vi "AcquisitionMVF_Reentrent.vi"(6 "error in":errorcluster, 7 "Session":T2, 9 "Image Rev":T1) -> (0 "camera error":errorcluster, 2 "Image Dst Out":T1, 3 "Acquisition OK?":bool)   [LabVIEW 2011]
uses:
  <vilib>/vision/Image Controls.llb/IMAQ Image.ctl
  <vilib>/userdefined/High Color/IMAQdx.ctl
  <vilib>/vision/NI_Vision_Development_Module.lvlib
  <vilib>/vision/driver/NI_Vision_Acquisition_Software.lvlib
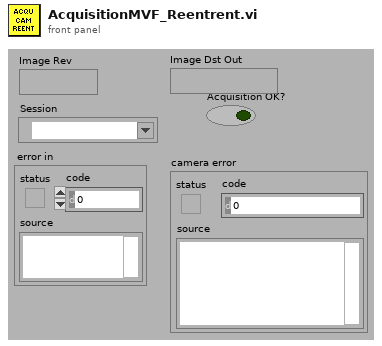
[diagram p1: front panel]
types:
  T1 = typedef "IMAQ Image.ctl" = refnum<image>
  T2 = typedef "IMAQdx.ctl" = refnum<k21>
  T3 = typedef "Image Type" = u32
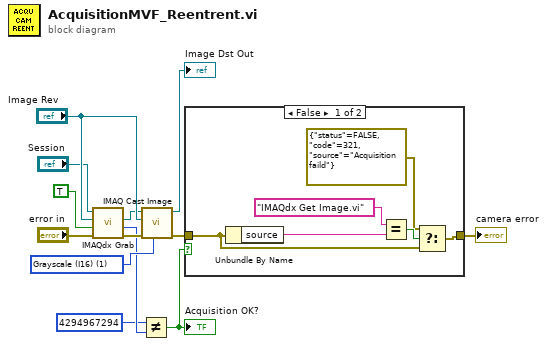
[diagram p0: block diagram]
diagram:
  w7 = T3 1 items=["Grayscale (U8)", "Grayscale (I16)", "Grayscale (SGL)", "Complex (CSG)", "RGB (U32)", "HSL (U32)", "RGB (U64)", "Grayscale (U16)"] ("Image Type")
  n1 = call <vilib>:"IMAQdx Grab.vi"("error in"="error in", "Wait for Next Buffer? (Yes)"=TRUE, "Image In"="Image Rev", "Session In"="Session") -> ("error out"=w6:errorcluster, "Buffer Number Out"=w3:u32, "Image Out"=w8:T1)  [unwired: 5 out]
  n2 = Not Equal?(x=u32 4294967294 ("Buffer Number Out"), y=w3) -> (x != y?=w13:bool)
  "Acquisition OK?" <- w13
  n3 = call "IMAQ Cast Image"("Image Type"=w7, "error in (no error)"=w6, "Image Dst"="Image Rev", "Image Src"=w8) -> ("error out"=w5:errorcluster, "Image Dst Out"=→"Image Dst Out":T1)  [unwired: 6 in]
  n4 = case shown="False" w13 {
    tunnel: w5 -> [w15 w20]
    tunnel: [w14 w20] -> w9
    frame False {
      n5 = Unbundle By Name(w15) -> ("source"=w19:string)
      n6 = Equal?(x="IMAQdx Get Image.vi", y=w19) -> (x = y?=w17:bool)
      n7 = Select(t=errorcluster {"status"=FALSE, "code"=321, "source"="Acquisition faild"} ("error in"), s=w17, f=w15) -> (s? t:f=w14:errorcluster)
    }
    frame True {
    }
  }
  "camera error" <- w9
